vi "Timer Interupt Example.vi"   [LabVIEW 2014]
uses:
  <vilib>/Aledyne-TSXperts/Arduino Compatible Compiler for LabVIEW/Code Generator/Arduino APIs/Digital/PinDirection.ctl
  <vilib>/Aledyne-TSXperts/Arduino Compatible Compiler for LabVIEW/Arduino Compatible Compiler for LabVIEW.lvlib
  QwaveSys_ESP8266/QwaveSys_ESP8266.lvlib
types:
  T1 = typedef "Arduino Compatible Compiler for LabVIEW.lvlib/PinDirection.ctl" = enum16{" INPUT", "OUTPUT", " INPUT_PULLUP"}
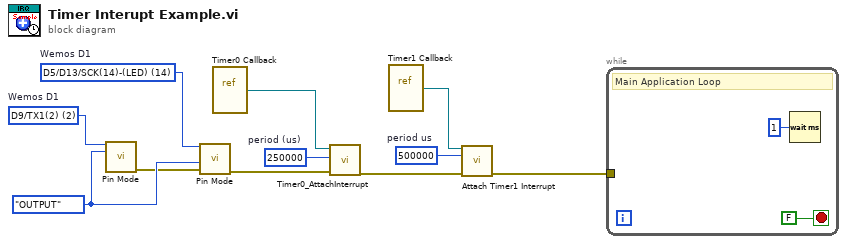
[diagram p0: block diagram]
diagram:
  w2 = u8 2 items=["D0-RX(3)"=3, "D1-TX(1)"=1, "D2(16)"=16, "D3/D15/SCL(5)"=5, "D4/D14/SDA(4)"=4, "D5/D13/SCK(14)-(LED)"=14, "D6/D12/MISO(12)"=12, "D7/D11/MOSI(13)"=13, "D8(0)"=0, "D9/TX1(2)"=2, "D10/SS (15)"=15, "ADC0,(17)"=17]  # Wemos D1
  w1 = u8 14 items=["D0-RX(3)"=3, "D1-TX(1)"=1, "D2(16)"=16, "D3/D15/SCL(5)"=5, "D4/D14/SDA(4)"=4, "D5/D13/SCK(14)-(LED)"=14, "D6/D12/MISO(12)"=12, "D7/D11/MOSI(13)"=13, "D8(0)"=0, "D9/TX1(2)"=2, "D10/SS (15)"=15, "ADC0,(17)"=17]  # Wemos D1
  w8 = PinDirection."OUTPUT" ("direction")
  w9 = u32 500000  # period us
  w3 = u32 250000  # period (us)
  n1 = call <vilib>:"Pin Mode.vi"("pin"=w2, "direction"=w8) -> ("error out"=w7:errorcluster)  [unwired: 13 in]
  n2 = call <vilib>:"Pin Mode.vi"("pin"=w1, "direction"=w8, "error in (no error)"=w7) -> ("error out"=w6:errorcluster)  [unwired: 12 in]
  n3 = vi-ref "Timer0 Callback.vi"() -> (w4:refnum<vi>)
  n4 = call "Timer0_AttachInterrupt.vi"("error in (no error)"=w6, "period (us)"=w3, "VI Reference"=w4) -> ("error out"=w5:errorcluster)  [unwired: 8 in]
  n5 = vi-ref "Timer1 Callback.vi"() -> (w10:refnum<vi>)
  n6 = call <vilib>:"Attach Timer1 Interrupt.vi"("VI Reference"=w10, "period"=w9, "error in (no error)"=w5) -> ("error out"=w11:errorcluster)  [unwired: 12 in]
  n7 = while {
    tunnel: w11 -> [_]
    stop <- FALSE stop-if-true
    # "Main Application Loop"
    n8 = Wait (ms)(milliseconds to wait=u32 1) -> ()  [unwired: 1 out]
  }
